vi "lvToUnixTime.vi"(8 "error in":errorcluster, 11 "Local Time Stamp":timestamp) -> (0 "error out":errorcluster, 3 "Unix Time (in milliseconds)":u64)   [LabVIEW 2013, in "ProcessInfo.lvlib"]
uses:
  ProcessInfo.lvlib
  <vilib>/Utility/miscctls.llb/LVDateTimeRec.ctl
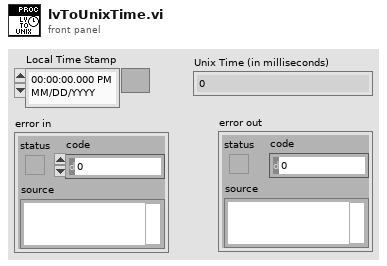
[diagram p1: front panel]
types:
  T1 = typedef "LVDateTimeRec.ctl" = cluster{"fractional second":dbl, "second":i32, "minute":i32, "hour":i32, "day of month":i32, "month":i32, "year":i32, "day of week":i32, "day of year":i32, "DST":i32}
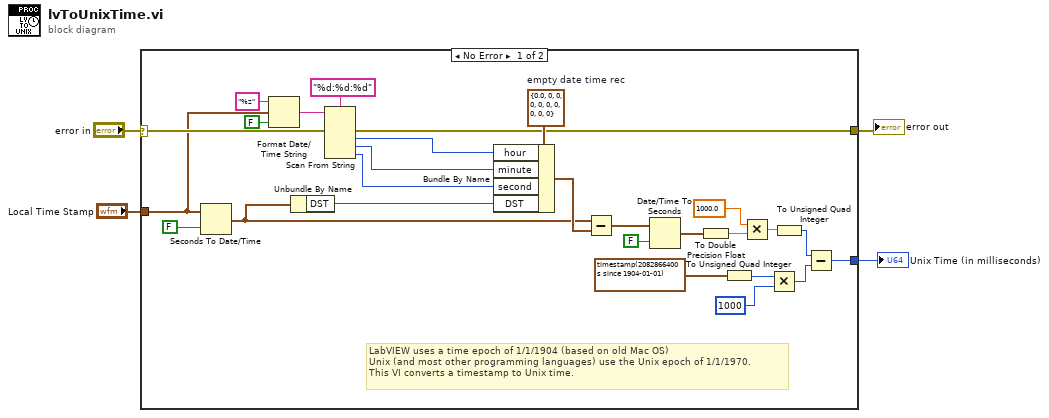
[diagram p0: block diagram]
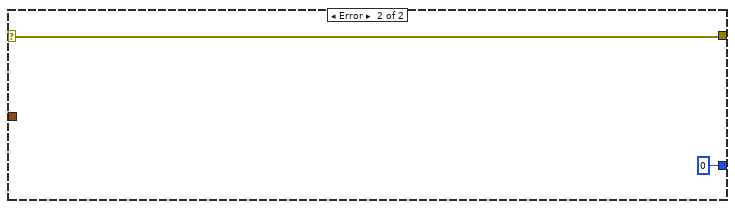
[diagram p2: hidden frame]
diagram:
  n1 = case shown="No Error" "error in" {
    selector: "error in" -> [w10 w33]
    tunnel: "Local Time Stamp" -> [w8 _]
    tunnel: [w21 u64 0] -> w2
    tunnel: [w9 w33] -> w3
    frame No Error {
      w27 = T1 {"fractional second"=0.0, "second"=0, "minute"=0, "hour"=0, "day of month"=0, "month"=0, "year"=0, "day of week"=0, "day of year"=0, "DST"=0}  # empty date time rec
      # "LabVIEW uses a time epoch of 1/1/1904 (based on old Mac OS)\nUnix (and most other programming languages) use the Unix epoch of 1/1/1970.\nThis VI converts a timestamp to Unix time."
      n2 = Seconds To Date/Time(time stamp (now)=w8, to UTC (F)=FALSE) -> (date time rec=w6:T1)
      n3 = Format Date/Time String(time format string (%c)="%z", seconds (now)=w8, UTC format=FALSE) -> (date/time string=w30:string)
      n4 = Unbundle By Name(w6) -> ("DST"=w5:i32)
      n5 = Scan From String(format string="%d:%d:%d", input string=w30, error in=w10) -> (error out=w9:errorcluster, output 1=w7:i32, output 2=w28:i32, output 3=w29:i32)  [unwired: 4 in, 2 out]
      n6 = Bundle By Name(cluster=w27, "hour"=w7, "minute"=w28, "second"=w29, "DST"=w5) -> (w23:T1)
      n7 = Subtract(x=w6, y=w23) -> (x-y=w24:T1)
      n8 = Date/Time To Seconds(1:FALSE ("is UTC (F)"), 2:w24) -> (0:w18:timestamp)
      n9 = To Double Precision Float(number=w18) -> (double precision float=w16:dbl)
      n10 = To Unsigned Quad Integer(1:timestamp(2082866400 s since 1904-01-01) ("time stamp")) -> (0:w15:u64)
      n11 = Multiply(x=1000.0, y=w16) -> (x*y=w13:dbl)
      n12 = Multiply(x=w15, y=u64 1000) -> (x*y=w11:u64)
      n13 = To Unsigned Quad Integer(1:w13) -> (0:w12:u64)
      n14 = Subtract(x=w12, y=w11) -> (x-y=w21:u64)
    }
    frame Error {
    }
  }
  "Unix Time (in milliseconds)" <- w2
  "error out" <- w3
